vi "McPherson get status.vi"(4 "Status":T1(ring)=enum."Full (X, ^, Z0)", 5 "error in (no error)":errorcluster, 7 "Wait(ms)":u32=50, 8 "VISA Resource Name":refnum<visa-resource-name>) -> (0 "error out":errorcluster, 1 "CurrentPosition":i32, 2 "StatusParameter":T2={"StepperPosition"=0, "MovingStatus"=0, "V"=42372, "K"=5, "I"=30341}, 3 "dup VISA Resource Name":refnum<visa-resource-name>)   [LabVIEW 2019]
uses:
  Serial Instruments/Serial Support VISA.llb/Serial Actions.ctl
  Globals and TypeDefs/Error Categories.ctt
  <vilib>/Utility/error.llb/DialogType.ctl
  Globals and TypeDefs/gSpectrometer.vi
panel:
  out "MovingStatus":i32
  out "Initial Velocity I":i32=30341
  out "Ramp Factor K":i32=5
  out "Velocity (Steps/s)":i32=42372
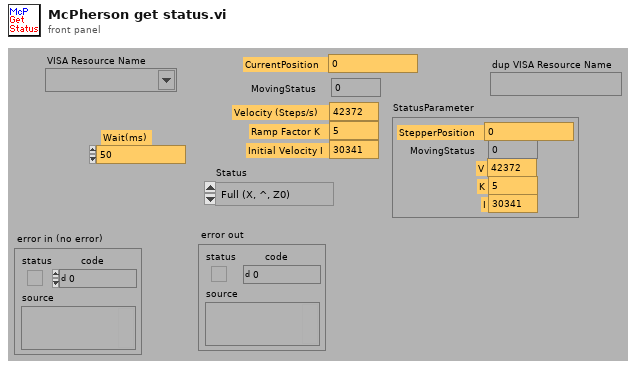
[diagram p1: front panel]
types:
  T1 = enum16{"Grab Globals", "Full (X, ^, Z0)", "Moving(^ and Z0)", "Position(Z0)"}
  T2 = cluster{"StepperPosition":i32, "MovingStatus":i32, "V":i32, "K":i32, "I":i32}
  T3 = typedef "Serial Actions.ctl" = enum16{"Init", "Break", "Clear Buffer", "Write", "Read", "N Bytes", "Lock", "Unlock", "Close"}
  T4 = enum8{"Initialization Error", "Command Error", "Parameter Error", "Overflow Error", "Time-out Error", "Misc Error", "User cancel"}
  T5 = typedef "Error Categories.ctt" = enum8{"General", "CCD-256x1024", "CCD-1340x400", "InGaAs PDA", "McPherson 2075", "Magnetic Field", "Temperature Control", "Other"}
  T6 = cluster{"CurrentStepperPosition":i32, "offset (0)":i32, "McP Scan Velocity":i32, i32, i32}
  T7 = typedef "DialogType.ctl" = u16
  T8 = cluster{i32, i32, "McP Scan Velocity":i32, i32, i32}
  T9 = cluster{i32, "offset (0)":i32, "McP Scan Velocity":i32, i32, i32}
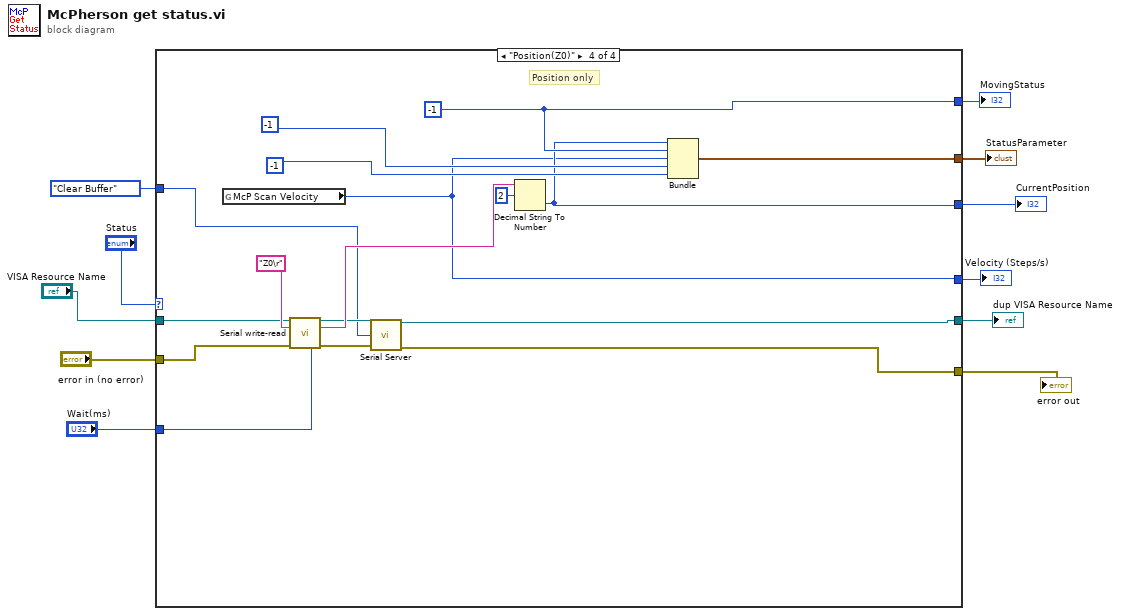
[diagram p0: block diagram]
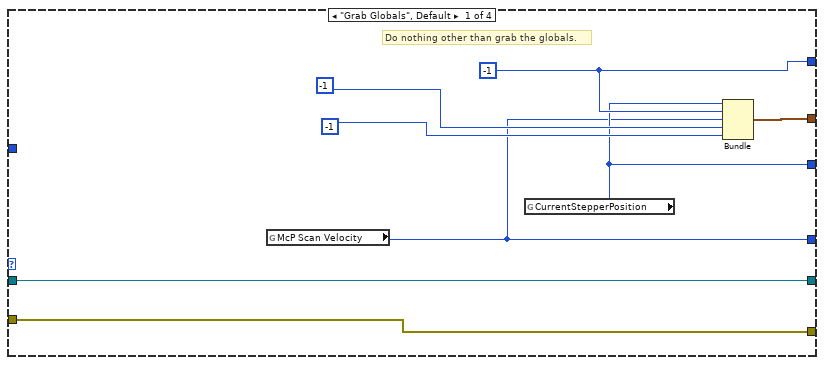
[diagram p2: hidden frame]
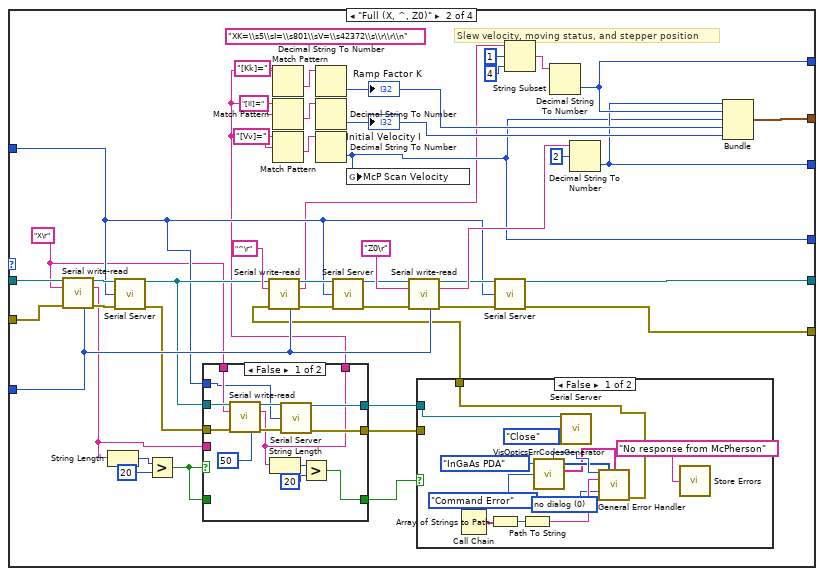
[diagram p3: hidden frame]
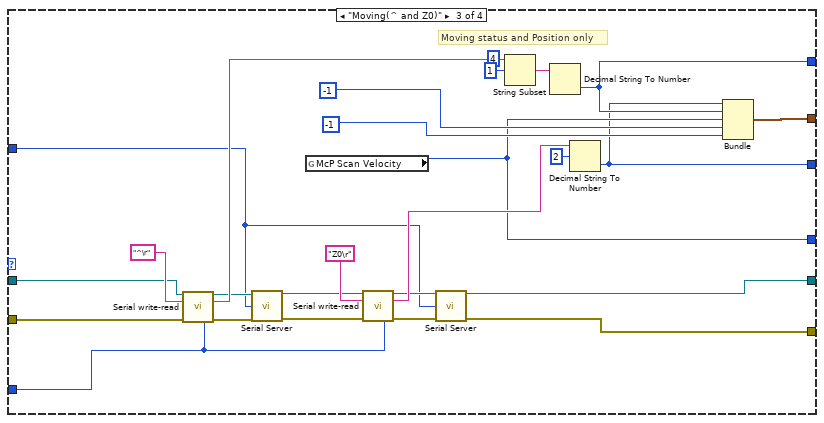
[diagram p6: hidden frame]
diagram:
  n1 = case shown="\"Position(Z0)\"" "Status" {
    tunnel: [w15 w35 w100 w126] -> w11
    tunnel: "error in (no error)" -> [w15 w60 w110 w132]
    tunnel: [w19 w49 w114 w136] -> w2
    tunnel: "VISA Resource Name" -> [w14 w44 w109 w130]
    tunnel: "Wait(ms)" -> [_ w46 w104 w131]
    tunnel: [w16 w45 w111 w133] -> w8
    tunnel: [w13 w22 w97 w124] -> w1
    tunnel: [w12 w21 w98 w123] -> w7
    tunnel: [w14 w34 w99 w125] -> w4
    tunnel: Serial_Actions."Clear Buffer" ("Action") -> [_ w31 w101 w127]
    frame "Grab Globals", Default {
      w16 = -1 ("offset (0)")
      # "Do nothing other than grab the globals."
      n2 = global read "gSpectrometer.vi" "McP Scan Velocity"() -> (w12:i32)
      n3 = global read "gSpectrometer.vi" "CurrentStepperPosition"() -> (w13:i32)
      n4 = Bundle("CurrentStepperPosition"=w13, "offset (0)"=w16, "McP Scan Velocity"=w12, -1, -1) -> (w19:T6)  [unwired: 1 in]
    }
    frame "Full (X, ^, Z0)" {
      (unwired) "XK=\\s5\\sI=\\s801\\sV=\\s42372\\s\\r\\r\\n"
      w29 = "X\r" ("String To Send")
      # "Slew velocity, moving status, and stepper position"
      n5 = call "Serial write-read.vi"("VISA Resource Name"=w44, "String To Send"=w29, "error in (no error)"=w60, "milliseconds to wait"=w46) -> ("dup VISA Resource Name"=w42:refnum<visa-resource-name>, "Serial Read"=w30:string, "error out"=w43:errorcluster)  [unwired: 6 in, 3 out]
      n6 = String Length(string=w30) -> (length=w63:i32)
      n7 = call "Serial Server.vi"("VISA Resource Name"=w42, "Action"=w31, "error in (no error)"=w43) -> ("dup VISA Resource Name"=w32:refnum<visa-resource-name>, "error out"=w33:errorcluster)  [unwired: 8 in, 3 out]
      n8 = Greater?(x=w63, y=20) -> (0:w28:bool)
      n9 = case shown="False" w28 {
        tunnel: w33 -> [w78 w81]
        tunnel: w32 -> [w77 w80]
        tunnel: w31 -> [w73 _]
        tunnel: w29 -> [w76 _]
        tunnel: [w70 w82] -> w26
        tunnel: w28 -> [_ w82]
        tunnel: [w69 w81] -> w25
        tunnel: [w68 w80] -> w23
        tunnel: w30 -> [_ w79]
        tunnel: [w66 w79] -> w27
        frame False {
          n10 = call "Serial write-read.vi"("VISA Resource Name"=w77, "String To Send"=w76, "error in (no error)"=w78, "milliseconds to wait"=u32 50) -> ("dup VISA Resource Name"=w74:refnum<visa-resource-name>, "Serial Read"=w66:string, "error out"=w75:errorcluster)  [unwired: 6 in, 3 out]
          n11 = String Length(string=w66) -> (length=w72:i32)
          n12 = call "Serial Server.vi"("VISA Resource Name"=w74, "Action"=w73, "error in (no error)"=w75) -> ("dup VISA Resource Name"=w68:refnum<visa-resource-name>, "error out"=w69:errorcluster)  [unwired: 8 in, 3 out]
          n13 = Greater?(x=w72, y=20) -> (0:w70:bool)
        }
        frame True {
        }
      }
      n14 = Match Pattern(string=w27, regular expression="[Kk]=") -> (after substring=w57:string)  [unwired: 1 in, 3 out]
      n15 = Match Pattern(string=w27, regular expression="[Ii]=") -> (after substring=w58:string)  [unwired: 1 in, 3 out]
      n16 = Match Pattern(string=w27, regular expression="[Vv]=") -> (after substring=w59:string)  [unwired: 1 in, 3 out]
      n17 = Decimal String To Number(string=w57) -> (number=w48:i32)  [unwired: 2 in, 1 out]
      "Ramp Factor K" <- w48
      n18 = Decimal String To Number(string=w58) -> (number=w47:i32)  [unwired: 2 in, 1 out]
      "Initial Velocity I" <- w47
      n19 = Decimal String To Number(string=w59) -> (number=w21:i32)  [unwired: 2 in, 1 out]
      n20 = global write "gSpectrometer.vi" "McP Scan Velocity"(w21) -> ()
      n21 = case shown="False" w26 {
        tunnel: w25 -> [_ w96]
        tunnel: [w83 w96] -> w24
        tunnel: w23 -> [w94 _]
        frame False {
          w84 = T7 0 items=["no dialog", "OK message", "continue or stop message", "OK message + warnings", "continue/stop + warnings"] ("type of dialog (OK msg:1)")
          n22 = Call Chain() -> (call chain=w90:string[])
          n23 = Array of Strings to Path(0:w90) -> (2:w91:path)  [unwired: 1 in]
          n24 = Path To String(path=w91) -> (string=w92:string)
          n25 = call "VisOpticsErrCodesGenerator.vi"("NHMFL Visible Optics Error Type"=T4."Command Error", "NHMFL Visible Optics Error Categories"=Error_Categories.ctt."InGaAs PDA") -> ("user-defined descriptions"=w85:string[], "User-defined Error Code"=w89:i32, "user-defined codes"=w86:i32[])  [unwired: 1 in, 3 out]
          n26 = call "Serial Server.vi"("VISA Resource Name"=w94, "Action"=Serial_Actions."Close") -> ()  [unwired: 9 in, 5 out]
          n27 = call <vilib>:"General Error Handler.vi"("[error code] (0)"=w89, "[user-defined codes]"=w86, "[user-defined descriptions]"=w85, "[error source] (\" \")"=w92, "type of dialog (OK msg:1)"=w84) -> ("error out"=w83:errorcluster)  [unwired: 6 in, 4 out]
          n28 = call "Store Errors.vi"("New Error"="No response from McPherson") -> ()  [unwired: 1 in]
        }
        frame True {
        }
      }
      n29 = call "Serial write-read.vi"("VISA Resource Name"=w32, "String To Send"="^\r", "error in (no error)"=w24, "milliseconds to wait"=w46) -> ("dup VISA Resource Name"=w40:refnum<visa-resource-name>, "Serial Read"=w20:string, "error out"=w41:errorcluster)  [unwired: 6 in, 3 out]
      n30 = call "Serial Server.vi"("VISA Resource Name"=w40, "Action"=w31, "error in (no error)"=w41) -> ("dup VISA Resource Name"=w38:refnum<visa-resource-name>, "error out"=w39:errorcluster)  [unwired: 8 in, 3 out]
      n31 = call "Serial write-read.vi"("VISA Resource Name"=w38, "String To Send"="Z0\r", "error in (no error)"=w39, "milliseconds to wait"=w46) -> ("dup VISA Resource Name"=w36:refnum<visa-resource-name>, "Serial Read"=w61:string, "error out"=w37:errorcluster)  [unwired: 6 in, 3 out]
      n32 = call "Serial Server.vi"("VISA Resource Name"=w36, "Action"=w31, "error in (no error)"=w37) -> ("dup VISA Resource Name"=w34:refnum<visa-resource-name>, "error out"=w35:errorcluster)  [unwired: 8 in, 3 out]
      n33 = String Subset(string=w20, offset (0)=1, length (rest)=4) -> (substring=w52:string)
      n34 = Decimal String To Number(string=w52) -> (number=w45:i32)  [unwired: 2 in, 1 out]
      n35 = Decimal String To Number(string=w61, offset=2) -> (number=w22:i32)  [unwired: 1 in, 1 out]
      n36 = Bundle(w22, w45, w21, w48, w47) -> (w49:cluster{i32, i32, i32, i32, i32})  [unwired: 1 in]
    }
    frame "Moving(^ and Z0)" {
      # "Moving status and Position only"
      n37 = call "Serial write-read.vi"("VISA Resource Name"=w109, "String To Send"="^\r", "error in (no error)"=w110, "milliseconds to wait"=w104) -> ("dup VISA Resource Name"=w107:refnum<visa-resource-name>, "Serial Read"=w119:string, "error out"=w108:errorcluster)  [unwired: 6 in, 3 out]
      n38 = call "Serial Server.vi"("VISA Resource Name"=w107, "Action"=w101, "error in (no error)"=w108) -> ("dup VISA Resource Name"=w105:refnum<visa-resource-name>, "error out"=w106:errorcluster)  [unwired: 8 in, 3 out]
      n39 = global read "gSpectrometer.vi" "McP Scan Velocity"() -> (w98:i32)
      n40 = call "Serial write-read.vi"("VISA Resource Name"=w105, "String To Send"="Z0\r", "error in (no error)"=w106, "milliseconds to wait"=w104) -> ("dup VISA Resource Name"=w102:refnum<visa-resource-name>, "Serial Read"=w120:string, "error out"=w103:errorcluster)  [unwired: 6 in, 3 out]
      n41 = call "Serial Server.vi"("VISA Resource Name"=w102, "Action"=w101, "error in (no error)"=w103) -> ("dup VISA Resource Name"=w99:refnum<visa-resource-name>, "error out"=w100:errorcluster)  [unwired: 8 in, 3 out]
      n42 = String Subset(string=w119, offset (0)=1, length (rest)=4) -> (substring=w117:string)
      n43 = Decimal String To Number(string=w117) -> (number=w111:i32)  [unwired: 2 in, 1 out]
      n44 = Decimal String To Number(string=w120, offset=2) -> (number=w97:i32)  [unwired: 1 in, 1 out]
      n45 = Bundle(w97, w111, "McP Scan Velocity"=w98, -1, -1) -> (w114:T8)  [unwired: 1 in]
    }
    frame "Position(Z0)" {
      w133 = -1 ("offset (0)")
      # "Position only"
      n46 = global read "gSpectrometer.vi" "McP Scan Velocity"() -> (w123:i32)
      n47 = call "Serial write-read.vi"("VISA Resource Name"=w130, "String To Send"="Z0\r", "error in (no error)"=w132, "milliseconds to wait"=w131) -> ("dup VISA Resource Name"=w128:refnum<visa-resource-name>, "Serial Read"=w138:string, "error out"=w129:errorcluster)  [unwired: 6 in, 3 out]
      n48 = call "Serial Server.vi"("VISA Resource Name"=w128, "Action"=w127, "error in (no error)"=w129) -> ("dup VISA Resource Name"=w125:refnum<visa-resource-name>, "error out"=w126:errorcluster)  [unwired: 8 in, 3 out]
      n49 = Decimal String To Number(string=w138, offset=2) -> (number=w124:i32)  [unwired: 1 in, 1 out]
      n50 = Bundle(w124, "offset (0)"=w133, "McP Scan Velocity"=w123, -1, -1) -> (w136:T9)  [unwired: 1 in]
    }
  }
  "error out" <- w11
  "StatusParameter" <- w2
  "MovingStatus" <- w8
  "CurrentPosition" <- w1
  "Velocity (Steps/s)" <- w7
  "dup VISA Resource Name" <- w4
